vi "SGUI Assign Multiple Strings With Tags By Label.vi"(6 "error in":errorcluster, 8 "label(s) (empty)":string, 9 "string (empty)":string, 10 "keep last font face setup (False)":bool) -> (7 "error out":errorcluster, 11 "control references out":refnum<vi>[](array[refnum]))   [LabVIEW 2020, in "varilib.lvlib"]
doc: "This is multiline version of tag formatted text writter. The destination string objects are pointed by label string(s). If multiple string objects are assigned a multiline string with labels is entered to 'label(s)' input. When more than one label is entered the 'string' is parsed into lines. Each line is assigned to one of the referenced string objects. If there are more lines of text than references the rest of the 'string' is assigned to the last referenced string object.\n\nFor format details see single string object function.\n\nKeep in mind the format tags applies always only for one line (one referenced string object). So when multiple lines are to have the same format the tags must be repeated for each line!\n\nThi VI ignores input errors (will execute anyway) however will generate error if any of the named controls is not found or writting to it fails (invalid type of control)."
uses:
  varilib.lvlib
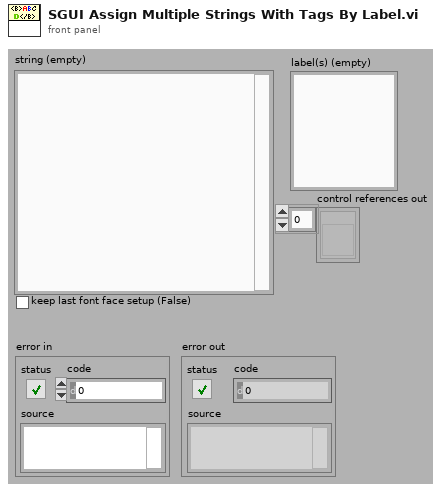
[diagram p1: front panel]
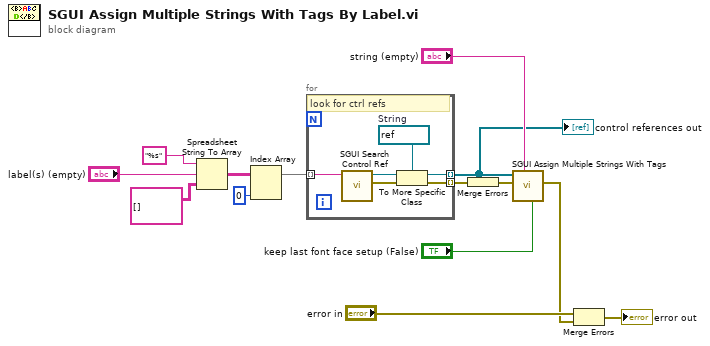
[diagram p0: block diagram]
diagram:
  n1 = Spreadsheet String To Array(format string="%s", spreadsheet string="label(s) (empty)", array type (2D Dbl)=string[][] []) -> (array=w12:string[][])  [unwired: 1 in]
  n2 = Index Array(array=w12, index (col)=0 ("disabled index (col)")) -> (element=w2:string[])  [unwired: 1 in]
  n3 = for {
    tunnel: w2 -> [w17] mode=indexing
    tunnel: [w16] -> w8 mode=indexing
    tunnel: [w15] -> w11 mode=indexing
    w18 = refnum<vi> refnum  # String
    # "look for ctrl refs"
    n4 = call "SGUI Search Control Ref.vi"("control label (empty)"=w17) -> ("error out"=w20:errorcluster, "control ref out"=w19:refnum<vi>)  [unwired: 8 in, 1 out]
    n5 = To More Specific Class(target class=w18, reference=w19, error in=w20) -> (specific class reference=w16:refnum<vi>, error out=w15:errorcluster)
  }
  "control references out" <- w8
  n6 = Merge Errors(w11) -> (w6:errorcluster)
  n7 = call "SGUI Assign Multiple Strings With Tags.vi"("error in"=w6, "string refs"=w8, "string (empty)"="string (empty)", "keep last font face setup (False)"="keep last font face setup (False)") -> ("error out"=w3:errorcluster)  [unwired: 6 in, 1 out]
  n8 = Merge Errors("error in", w3) -> (→"error out":errorcluster)
